vi "SetTempDir.vi"(8 "error in (no error)":errorcluster, 11 "SaveForPrevious in":refnum<class "SaveForPrevious.lvclass">) -> (0 "error out":errorcluster, 3 "SaveForPrevious out":refnum<class "SaveForPrevious.lvclass">)   [LabVIEW 2014, in "SaveForPrevious.lvclass"]
doc: "Sets versioned temporary path for downgrade."
uses:
  SaveForPrevious.lvclass
  SaveForPrevious.lvclass/SaveForPrevious.ctl
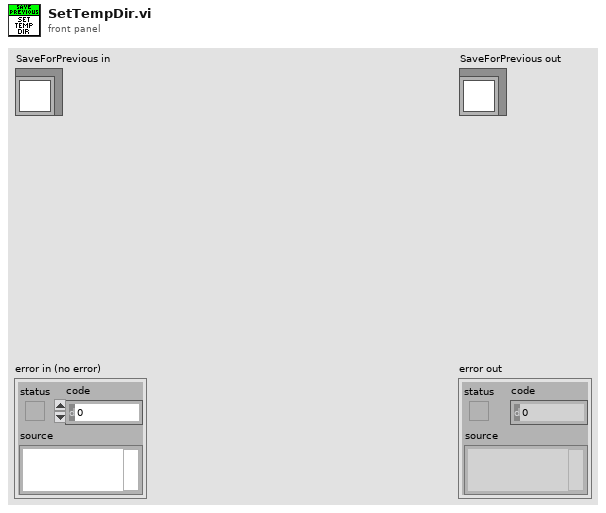
[diagram p1: front panel]
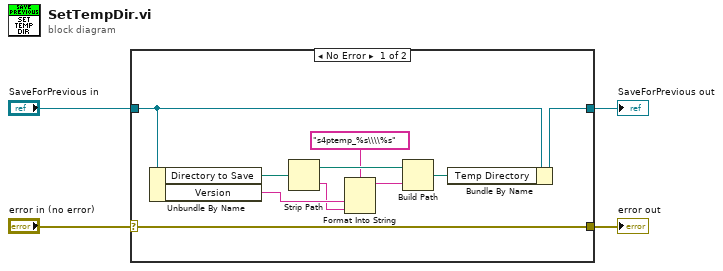
[diagram p0: block diagram]
diagram:
  n1 = case shown="No Error" "error in (no error)" {
    selector: "error in (no error)" -> [w14 w16]
    tunnel: [w14 w16] -> w3
    tunnel: [w5 w15] -> w1
    tunnel: "SaveForPrevious in" -> [w7 w15]
    frame No Error {
      n2 = Unbundle By Name(w7) -> ("Directory to Save"=w10:path, "Version"=w9:string)
      n3 = Strip Path(path=w10) -> (stripped path=w13:path, name=w8:string)
      n4 = Format Into String(format string="s4ptemp_%s\\\\%s", w9, w8) -> (resulting string=w11:string)  [unwired: 2 in, 1 out]
      n5 = Build Path(base path=w13, name or relative path=w11) -> (appended path=w6:path)
      n6 = Bundle By Name(cluster=w7, "Temp Directory"=w6) -> (w5:refnum<class "SaveForPrevious.lvclass">)
    }
    frame Error {
    }
  }
  "error out" <- w3
  "SaveForPrevious out" <- w1
